vi "SetPanelBackground.vi"(8 "error in (no error)":errorcluster, 11 "VI in":refnum<vi>) -> (0 "error out":errorcluster)   [LabVIEW 2024, in "Application.lvclass"]
uses:
  Application.lvclass
  Application.lvclass/Application.ctl
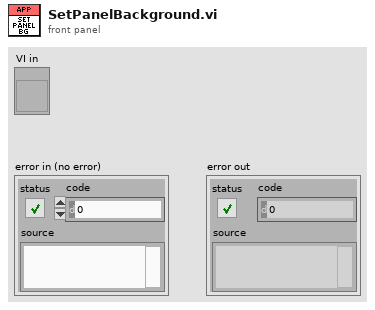
[diagram p1: front panel]
types:
  T1 = typedef "imagedata.ctl" = cluster{"image type":i32, "image depth":i32, "image":u8[], "mask":u8[], "colors":u32[], "Rectangle":cluster{"left":i16, "top":i16, "right":i16, "bottom":i16}}
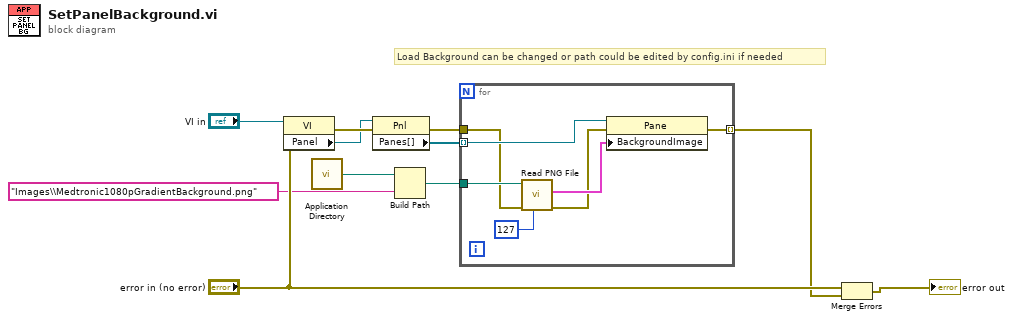
[diagram p0: block diagram]
diagram:
  # "Load Background can be changed or path could be edited by config.ini if needed"
  n1 = property class="VI"(reference="VI in", error in="error in (no error)") -> (error out=w7:errorcluster, "Panel"=w6:refnum<vi>)  [unwired: 1 out]
  n2 = call <vilib>:"Application Directory.vi"() -> ("Application Directory"=w4:path)
  n3 = property class="Pnl"(reference=w6, error in=w7) -> (error out=w9:errorcluster, "Panes[]"=w8:refnum<vi>[])  [unwired: 1 out]
  n4 = Build Path(base path=w4, name or relative path="Images\\Medtronic1080pGradientBackground.png") -> (appended path=w2:path)
  n5 = for {
    tunnel: w8 -> [w18] mode=indexing
    tunnel: w9 -> [w14]
    tunnel: [w17] -> w1 mode=indexing
    tunnel: w2 -> [w15]
    n6 = call <vilib>:"Read PNG File.vi"("Transparency Thresh"=u8 127, "error in (no error)"=w14, "path to PNG file"=w15) -> ("error out"=w13:errorcluster, "image data"=w16:T1)  [unwired: 6 in, 1 out]
    n7 = property class="Pane"(reference=w18, error in=w13, "BackgroundImage"=w16) -> (error out=w17:errorcluster)  [unwired: 1 out]
  }
  n8 = Merge Errors("error in (no error)", w1) -> (→"error out":errorcluster)
